vi "initialise variables.vi"(11 "messageHandler in":T1 {"params"."controlChannels"."ballControl" items=["Module6/output0", "Module6/output1", "Module6/output2", "Module6/output3", "Not-Used"]; "params"."controlChannels"."butterflyControl" items=["Module6/output0", "Module6/output1", "Module6/output2", "Module6/output3", "Not-Used"]; "params"."controlChannels"."speedControl" items=["Module6/output0", "Module6/output1", "Module6/output2", "Module6/output3", "Not-Used"]}) -> (3 "messageHandler out":T1 {"params"."controlChannels"."ballControl" items=["Module6/output0", "Module6/output1", "Module6/output2", "Module6/output3", "Not-Used"]; "params"."controlChannels"."butterflyControl" items=["Module6/output0", "Module6/output1", "Module6/output2", "Module6/output3", "Not-Used"]; "params"."controlChannels"."speedControl" items=["Module6/output0", "Module6/output1", "Module6/output2", "Module6/output3", "Not-Used"]})   [LabVIEW 2018]
uses:
  type defs/message handler data.ctl
  customVI/liveData/state.ctl
  Github/ICL-LabVIEW_General/data channels/parent class/channel type.ctl
  Github/ICL-LabVIEW_General/data channels/parent class/Supporting functions/channel filter - type.vi
  Github/ICL-LabVIEW_General/data channels/data channels.lvlib
  Github/ICL-LabVIEW_General/data channels/parent class/Data Channel.lvclass
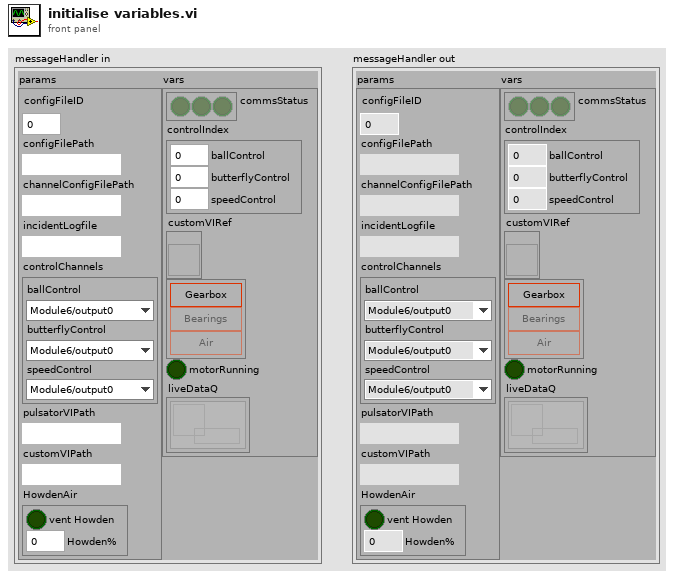
[diagram p1: front panel]
types:
  T1 = typedef "message handler data.ctl" = cluster{"params":cluster{"configFileID":u32, "configFilePath":path, "channelConfigFilePath":path, "incidentLogfile":path, "controlChannels":cluster{"ballControl":u16, "butterflyControl":u16, "speedControl":u16}, "pulsatorVIPath":path, "customVIPath":path, "HowdenAir":cluster{"vent Howden":bool, "Howden%":dbl}}, "vars":cluster{"commsStatus":bool[], "controlIndex":cluster{"ballControl":u16, "butterflyControl":u16, "speedControl":u16}, "customVIRef":refnum<vi>, "Interlocks":cluster{"gearboxOil":bool, "bearingOil":bool, "gearboxAir":bool}, "motorRunning":bool, "liveDataQ":refnum<queue>[]}}
  T2 = typedef "data channels.lvlib/Data Channel.lvclass/channel type.ctl" = enum16{"acquisition", "output", "other"}
  T3 = typedef "data channels.lvlib/Data Channel.lvclass/basic channel details.ctl" = cluster{"index":u16, "Active":bool, "channel name":string, "units":string, "module":string, "port":string, "liveOffset":dbl, "precision":u8, "channelType":T2, "fifoIndex":u16, "dataSource":T4, "acquireIndex":u16}
  T4 = typedef "data channels.lvlib/Data Channel.lvclass/dataSource.ctl" = enum16{"Not available", "FIFO", "Scanivalve", "Remote", "Calculated"}
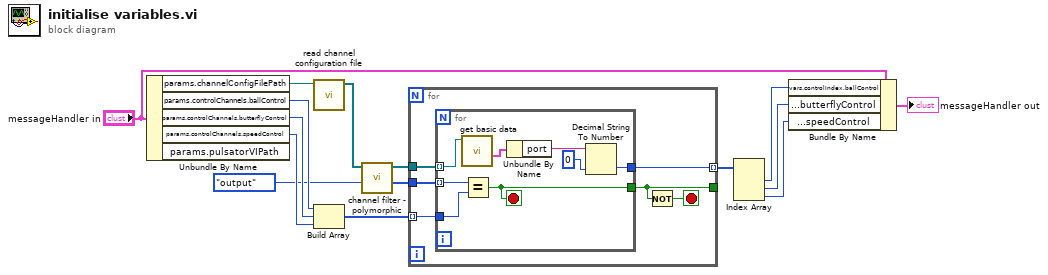
[diagram p0: block diagram]
diagram:
  n1 = Unbundle By Name("messageHandler in") -> ("params.channelConfigFilePath"=w9:path, "params.controlChannels.ballControl"=w13:u16, "params.controlChannels.butterflyControl"=w11:u16, "params.controlChannels.speedControl"=w12:u16)  [unwired: 1 out]
  n2 = call "read channel configuration file.vi"("config file"=w9) -> ("channelsArray"=w8:refnum<class "Data Channel.lvclass">[])  [unwired: 8 in, 2 out]
  n3 = Build Array(w13, w11, w12) -> (w10:u16[])
  n4 = call-poly "channel filter - polymorphic.vi"("channelType"=channel_type."output", "channels"=w8) -> ("filteredIndex"=w6:u16[], "filteredChannels"=w7:refnum<class "Data Channel.lvclass">[])  [unwired: 7 in, 1 out]
  n5 = for {
    tunnel: w7 -> [w21]
    tunnel: w10 -> [w20] mode=indexing
    tunnel: [w19] -> _
    tunnel: w6 -> [w17]
    tunnel: [w16] -> w5 mode=indexing
    stop <- w18 stop-if-true
    n6 = for {
      tunnel: w21 -> [w23] mode=indexing
      tunnel: w20 -> [w29]
      tunnel: [w28] -> w19
      tunnel: w17 -> [w27] mode=indexing
      tunnel: [w25] -> w16
      stop <- w28 stop-if-true
      n7 = call "get basic data.vi"("Data Channel in"=w23) -> ("details"=w22:T3)  [unwired: 9 in, 1 out]
      n8 = Equal?(x=w27, y=w29) -> (x = y?=w28:bool)
      n9 = Unbundle By Name(w22) -> ("port"=w26:string)
      n10 = Decimal String To Number(string=w26, default (0L)=u16 0 ("default (0 I32)")) -> (number=w25:u16)  [unwired: 1 in, 1 out]
    }
    n11 = Not(x=w19) -> (.not. x?=w18:bool)
  }
  n12 = Index Array(array=w5) -> (element #1=w4:u16, element #2=w3:u16, element #3=w2:u16)  [unwired: 3 in]
  n13 = Bundle By Name(cluster="messageHandler in", "vars.controlIndex.ballControl"=w4, "vars.controlIndex.butterflyControl"=w3, "vars.controlIndex.speedControl"=w2) -> (→"messageHandler out":T1)
